vi "ElevatorGlobal.vi"() -> ()   [LabVIEW 2023]
doc: "Arm global (getters and setter stuff)"
panel:
  out "Tune_Out_Min_Outer":dbl=0.03
  out "Tune_Out_Max_Outer":dbl=0.8
  out "Tune_Err_Thresh_Outer":dbl=7.5
  out "Tune_K_Grav_Outer":dbl
  out "ElevatorStage3LowWristClampActive":bool
  out "ElevatorStage3CmdSpecificHeight":dbl
  out "ElevatorStage3HighLimitSwitch":bool
  out "ElevatorStage3LowLimitSwitch":bool
  out "ElevatorStage3PosDemandHeight":dbl
  out "ElevatorStage3MotorOutput":dbl
  out "ElevatorStage3PositionHeight":dbl
  out "ElevatorOuterHighLimitSwitch":bool
  out "ElevatorOuterCmdSpecificHeight":dbl
  out "Tune_Out_Min":dbl=0.05
  out "Tune_Out_Max":dbl=1.0
  out "Tune_Err_Thresh":dbl=2.5
  out "Tune_K_Grav":dbl
  out "ElevatorOuterLowLimitSwitch":bool
  out "ElevatorExecOnTarget":bool
  out "ElevatorOuterPosDemandHeight":dbl
  out "ElevatorOuterMotorOutput":dbl
  out "ElevatorOuterPositionHeight":dbl
  # "#TODO Shoulder global rename globals --- maybe..."
  # "inner/stage 3 elevator motor globals"
  # "outer elevator motors globals"
  # "both"
  # "outer"
  # "inner"
  # "#TODO Once tuned, update these defaults with tuned values."
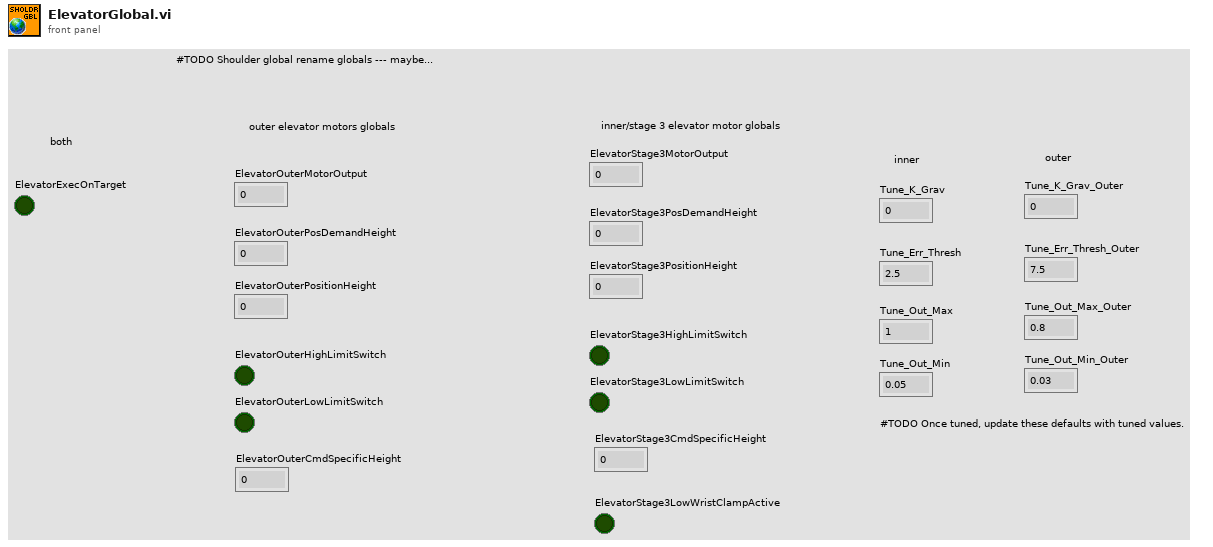
[diagram p1: front panel]
diagram:
